vi "Get Strings from Ref.vi"(8 "error in (no error)":errorcluster, 9 "Label Prefix":string, 10 "GObj Refnum in":refnum<vi>, 11 "StringControl in":refnum<class "StringControl.lvclass">) -> (0 "error out":errorcluster, 1 "Valid?":bool, 2 "GObj Refnum out":refnum<vi>, 3 "StringControl out":refnum<class "StringControl.lvclass">, 4 "GObj Name":string)   [LabVIEW 2013, in "SET Project Data.lvlib" / "StringControl.lvclass"]
uses:
  StringControl.lvclass
  Control/Control.lvclass
  GObject/GObject.lvclass
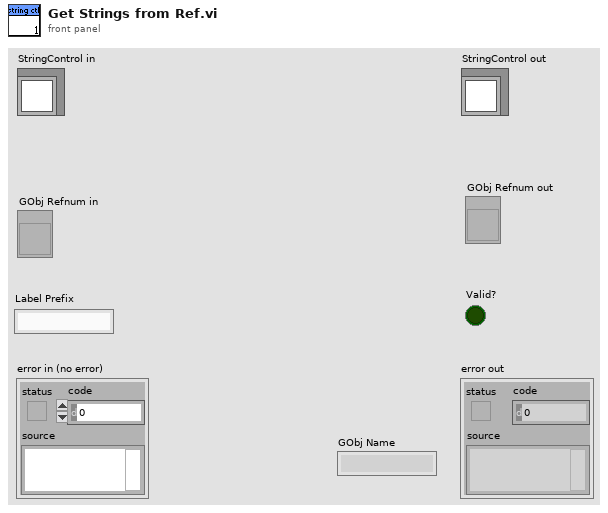
[diagram p1: front panel]
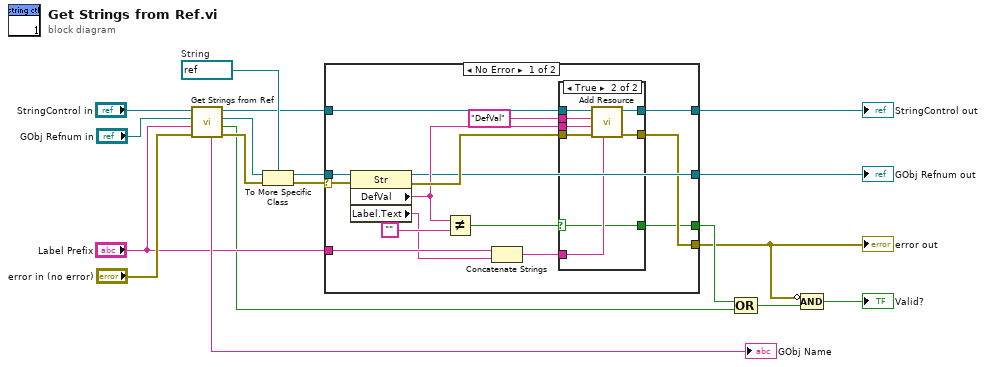
[diagram p0: block diagram]
diagram:
  w14 = refnum<vi> refnum  # String
  n1 = call-parent "Get Strings from Ref.vi"("error in (no error)"="error in (no error)", "Label Prefix"="Label Prefix", "GObj Refnum in"="GObj Refnum in", "Control in"="StringControl in") -> ("error out"=w12:errorcluster, "Valid?"=w5:bool, "GObj Refnum out"=w13:refnum<vi>, "Control out"=w10:refnum<class "StringControl.lvclass">, "GObj Name"=→"GObj Name":string)  [unwired: 3 in]
  n2 = To More Specific Class(target class=w14, reference=w13, error in=w12) -> (specific class reference=w11:refnum<vi>, error out=w8:errorcluster)
  n3 = case shown="No Error" w8 {
    selector: w8 -> [w29 w46]
    tunnel: w11 -> [w33 w45]
    tunnel: w10 -> [w31 w47]
    tunnel: [w30 w47] -> w9
    tunnel: [w25 w45] -> w7
    tunnel: "Label Prefix" -> [w24 _]
    tunnel: [w21 w46] -> w3
    tunnel: [w19 _] -> w4
    frame No Error {
      n4 = property class="Str"(reference=w33, error in=w29) -> (reference out=w25:refnum<vi>, error out=w28:errorcluster, "DefVal"=w26:string, "Label.Text"=w23:string)
      n5 = Not Equal?(x=w26, y="") -> (x != y?=w20:bool)
      n6 = Concatenate Strings(w24, w23) -> (w22:string)
      n7 = case shown="True" w20 {
        selector: w20 -> [w34 w37]
        tunnel: w31 -> [w36 w44]
        tunnel: [w36 w43] -> w30
        tunnel: w28 -> [w35 w42]
        tunnel: "DefVal" ("ItemName") -> [_ w41]
        tunnel: w26 -> [_ w40]
        tunnel: w22 -> [_ w39]
        tunnel: [w35 w38] -> w21
        tunnel: [w34 w37] -> w19
        frame False {
        }
        frame True {
          n8 = call "Add Resource.vi"("TagPrefix"=w39, "error in (no error)"=w42, "ItemText"=w40, "ItemName"=w41, "GObject in"=w44) -> ("error out"=w38:errorcluster, "GObject out"=w43:refnum<class "StringControl.lvclass">)  [unwired: 5 in]
        }
      }
    }
    frame Error {
    }
  }
  "error out" <- w3
  "StringControl out" <- w9
  "GObj Refnum out" <- w7
  n9 = Compound Arithmetic op=OR(w4, w5) -> (w2:bool)
  n10 = Compound Arithmetic op=AND(invert w3, w2) -> (→"Valid?":bool)
